vi "MHL_apply Savitzsky.vi"(0 "Data Cluster in":T1, 5 "error in (no error)":errorcluster) -> (14 "Data Cluster out":T1, 19 "error out":errorcluster)   [LabVIEW 2019, in "Main UI.lvlib"]
uses:
  Main UI.lvlib
  Module Data--cluster.ctl
  Neo-Laura-LVOOP/Class Library/XYgraph_class/XYgraph.lvclass
  FileReader/FPref_clustered--cluster references.ctl
  Main UI Shared/Boolean--FP cluster.ctl
  FileReader/FPref_cntrls--cluster references.ctl
  Main UI Shared/Indicators--FP cluster.ctl
  Analysis/Analysis.lvlib
  Main UI Shared/MAIN UI Shared.lvlib
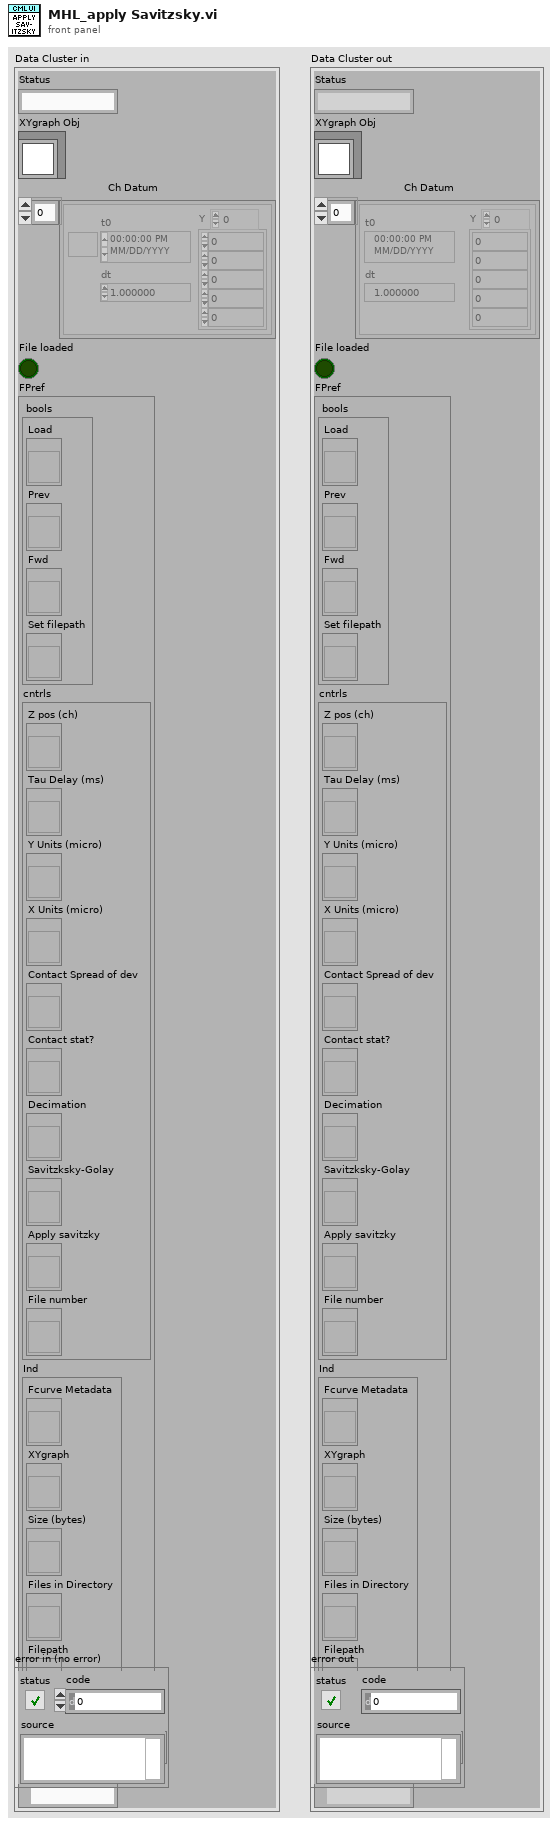
[diagram p1: front panel]
types:
  T1 = typedef "Main UI.lvlib/Module Data--cluster.ctl" = cluster{"Status":string, "XYgraph Obj":refnum<class "XYgraph.lvclass">, "Ch Datum":waveform(dbl)[], "File loaded":bool, "FPref":T2, "Tdms filepaths":path[], "TDMS filepath":path}
  T2 = typedef "FPref_clustered--cluster references.ctl" = cluster{" bools":T3, "cntrls":T4, "Ind":T5}
  T3 = typedef "MAIN UI Shared.lvlib/Boolean--FP cluster.ctl" = cluster{"Load":refnum<vi>, "Prev":refnum<vi>, "Fwd":refnum<vi>, "Set filepath":refnum<vi>}
  T4 = typedef "FPref_cntrls--cluster references.ctl" = cluster{"Z pos (ch)":refnum<vi>, "Tau Delay (ms)":refnum<vi>, "Y Units (micro)":refnum<vi>, "X Units (micro)":refnum<vi>, "Contact Spread of dev":refnum<vi>, "Contact stat?":refnum<vi>, "Decimation":refnum<vi>, "Savitzksky-Golay":refnum<vi>, "Apply savitzky ":refnum<vi>, "File number":refnum<vi>}
  T5 = typedef "Indicators--FP cluster.ctl" = cluster{"Fcurve Metadata":refnum<vi>, "XYgraph":refnum<vi>, "Size (bytes)":refnum<vi>, "Files in Directory":refnum<vi>, "Filepath":refnum<vi>}
  T6 = typedef "XYgraph.lvclass/Units --enum.ctl" = string
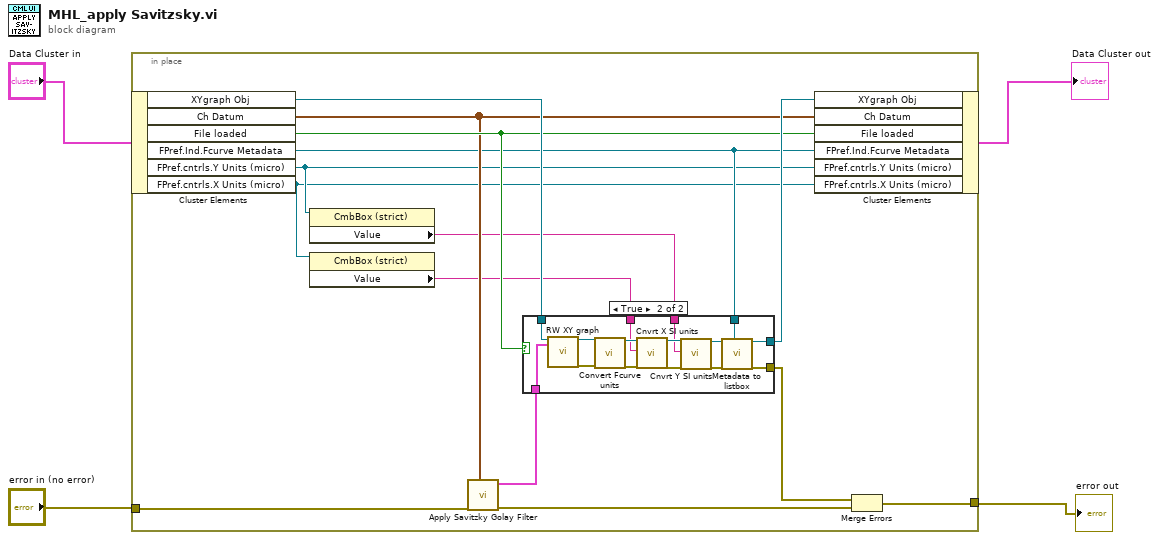
[diagram p0: block diagram]
diagram:
  n1 = in-place {
    in-place-border: "error in (no error)" -> [w15]
    in-place-border: [w10] -> w1
    n2 = in-place-cluster #1("Data Cluster in") -> ("XYgraph Obj"=w18:refnum<class "XYgraph.lvclass">, "Ch Datum"=w14:waveform(dbl)[], "File loaded"=w16:bool, "FPref.Ind.Fcurve Metadata"=w9:refnum<vi>, "FPref.cntrls.Y Units (micro)"=w8:refnum<vi>, "FPref.cntrls.X Units (micro)"=w7:refnum<vi>)
    n3 = property class="CmbBox (strict)"(reference=w8) -> ("Value"=w5:T6)  [unwired: 1 in, 2 out]
    n4 = property class="CmbBox (strict)"(reference=w7) -> ("Value"=w6:T6)  [unwired: 1 in, 2 out]
    n5 = call "Apply Savitzky Golay Filter.vi"("error in"=w15, "Ch Datum"=w14) -> ("error out"=w11:errorcluster, "Fcurve out"=w13:cluster{"X":dbl[], "Y":dbl[]}[])  [unwired: 7 in, 1 out]
    n6 = case shown="True" w16 {
      tunnel: w13 -> [_ w26]
      tunnel: w18 -> [w19 w25]
      tunnel: [w19 w24] -> w17
      tunnel: [_ w23] -> w12
      tunnel: w9 -> [_ w22]
      tunnel: w6 -> [_ w21]
      tunnel: w5 -> [_ w20]
      frame False {
      }
      frame True {
        n7 = call-dynamic "RW XY graph.vi"("reference in"=w25, "XY in"=w26) -> ("reference out"=w34:refnum<class "XYgraph.lvclass">, "error out"=w30:errorcluster)  [unwired: 15 in, 1 out]
        n8 = call-dynamic "Convert Fcurve units.vi"("reference in"=w34, "error in (no error)"=w30) -> ("reference out"=w31:refnum<class "XYgraph.lvclass">, "error out"=w29:errorcluster)  [unwired: 16 in]
        n9 = call-dynamic "Cnvrt X SI units.vi"("reference in"=w31, "X Units (micro)"=w21, "error in (no error)"=w29) -> ("reference out"=w33:refnum<class "XYgraph.lvclass">, "error out"=w32:errorcluster)  [unwired: 15 in]
        n10 = call-dynamic "Cnvrt Y SI units.vi"("reference in"=w33, "Units (micro)"=w20, "error in (no error)"=w32) -> ("reference out"=w28:refnum<class "XYgraph.lvclass">, "error out"=w27:errorcluster)  [unwired: 15 in]
        n11 = call-dynamic "Metadata to listbox.vi"("reference in"=w28, "error in (no error)"=w27, "Fcurve Metadata ref"=w22) -> ("reference out"=w24:refnum<class "XYgraph.lvclass">, "error out"=w23:errorcluster)  [unwired: 14 in, 1 out]
      }
    }
    n12 = in-place-cluster #1("XYgraph Obj"=w17, "Ch Datum"=w14, "File loaded"=w16, "FPref.Ind.Fcurve Metadata"=w9, "FPref.cntrls.Y Units (micro)"=w8, "FPref.cntrls.X Units (micro)"=w7) -> (→"Data Cluster out":T1)
    n13 = Merge Errors(w12, w11) -> (w10:errorcluster)
  }
  "error out" <- w1
